vi "Insert Key Value Pair (Single String).vi"(7 "key":string, 8 "error in (no error)":errorcluster, 10 "value":string, 11 "JSON Object in":refnum<class "JSON Value.lvclass">) -> (0 "error out":errorcluster, 1 "replaced":bool, 3 "JSON Object out":refnum<class "JSON Value.lvclass">)   [LabVIEW 2016, in "JSON Value.lvclass"]
uses:
  JSON Helper/JSON Value.lvclass
  JSON String/New JSON String.vi
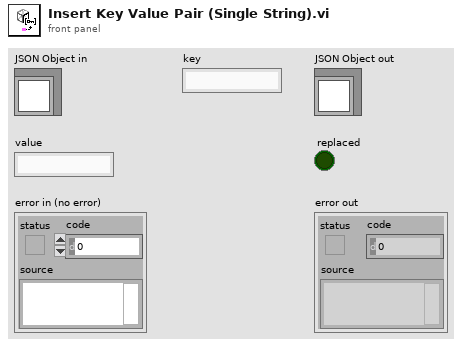
[diagram p1: front panel]
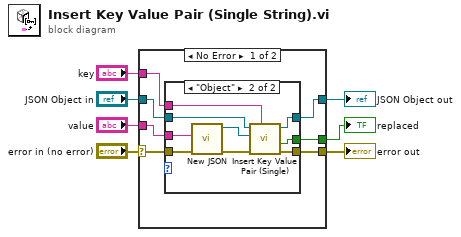
[diagram p0: block diagram]
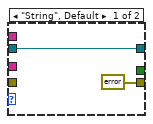
[diagram p2: hidden frame]
diagram:
  n1 = case shown="No Error" "error in (no error)" {
    selector: "error in (no error)" -> [w8 w27]
    tunnel: [w11 w27] -> w6
    tunnel: [w14 w26] -> w4
    tunnel: "JSON Object in" -> [w9 w26]
    tunnel: "key" -> [w13 _]
    tunnel: "value" -> [w12 _]
    tunnel: [w10 _] -> w1
    frame No Error {
      n2 = case shown="\"Object\"" {
        selector: _ -> [_ _]
        tunnel: [w16 w22] -> w14
        tunnel: w13 -> [_ w18]
        tunnel: w12 -> [_ w25]
        tunnel: [errorcluster {"status"=TRUE, "code"=-1000, "source"="Attempted insert on non-object"} ("error out") w19] -> w11
        tunnel: [_ w21] -> w10
        tunnel: w9 -> [w16 w23]
        tunnel: w8 -> [_ w24]
        frame "String", Default {
        }
        frame "Object" {
          n3 = call-poly "New JSON.vi"("error in (no error)"=w24, "value"=w25) -> ("error out"=w20:errorcluster, "JSON String out"=w17:refnum<class "JSON Value.lvclass">)  [unwired: 8 in]
          n4 = call "Insert Key Value Pair (Single).vi"("key"=w18, "error in (no error)"=w20, "JSON value"=w17, "JSON Object in"=w23) -> ("error out"=w19:errorcluster, "replaced"=w21:bool, "JSON Object out"=w22:refnum<class "JSON Value.lvclass">)  [unwired: 5 in]
        }
      }
    }
    frame Error {
    }
  }
  "error out" <- w6
  "JSON Object out" <- w4
  "replaced" <- w1
